vi "MSEncoder SubVI WfmCodeGen_PhaseScan.vi"(7 "Stepwise":i32, 8 "f2":ext, 9 "f1":ext, 10 "Scan time":ext, 11 "MSEncoder.lvclass":refnum<class "MSEncoder.lvclass">) -> (0 "WfmCode":u64[](array[numeric]), 1 "Actual Freq":dbl, 2 "Decyc":u64, 3 "1/Decyc":u32, 4 "error out":errorcluster)   [LabVIEW 2018, in "MSEncoder.lvclass"]
uses:
  MSEncoder.lvclass
  MSEncoder.lvclass/MSEncoder.ctl
panel:
  in  "High Res":bool
  in  "Interrupt":bool
  out "Phase Scan":cluster{"Scan time":ext, "Actual Freq":dbl}[](graph)
  out "Progress":dbl(slide) scale=0.0..0.05
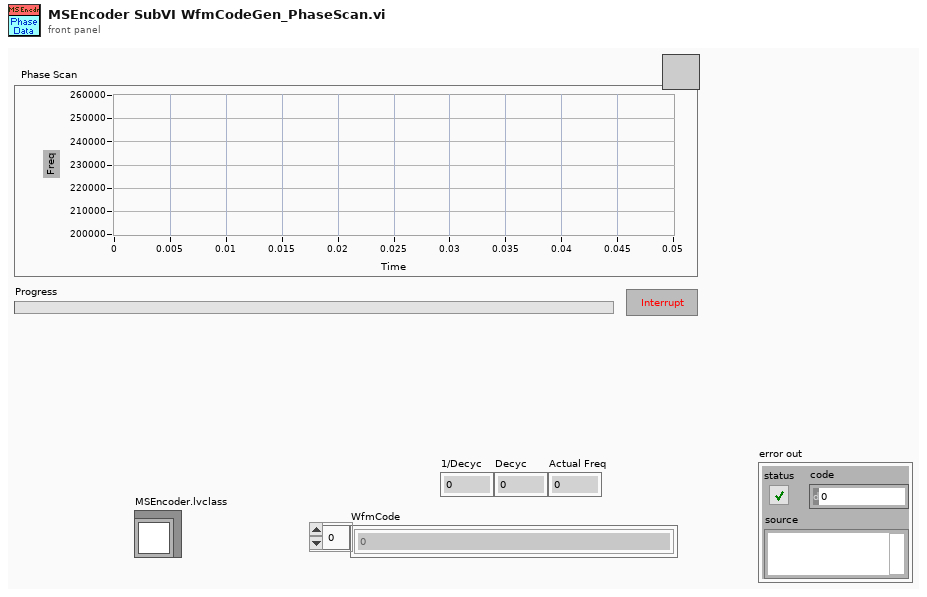
[diagram p1: front panel]
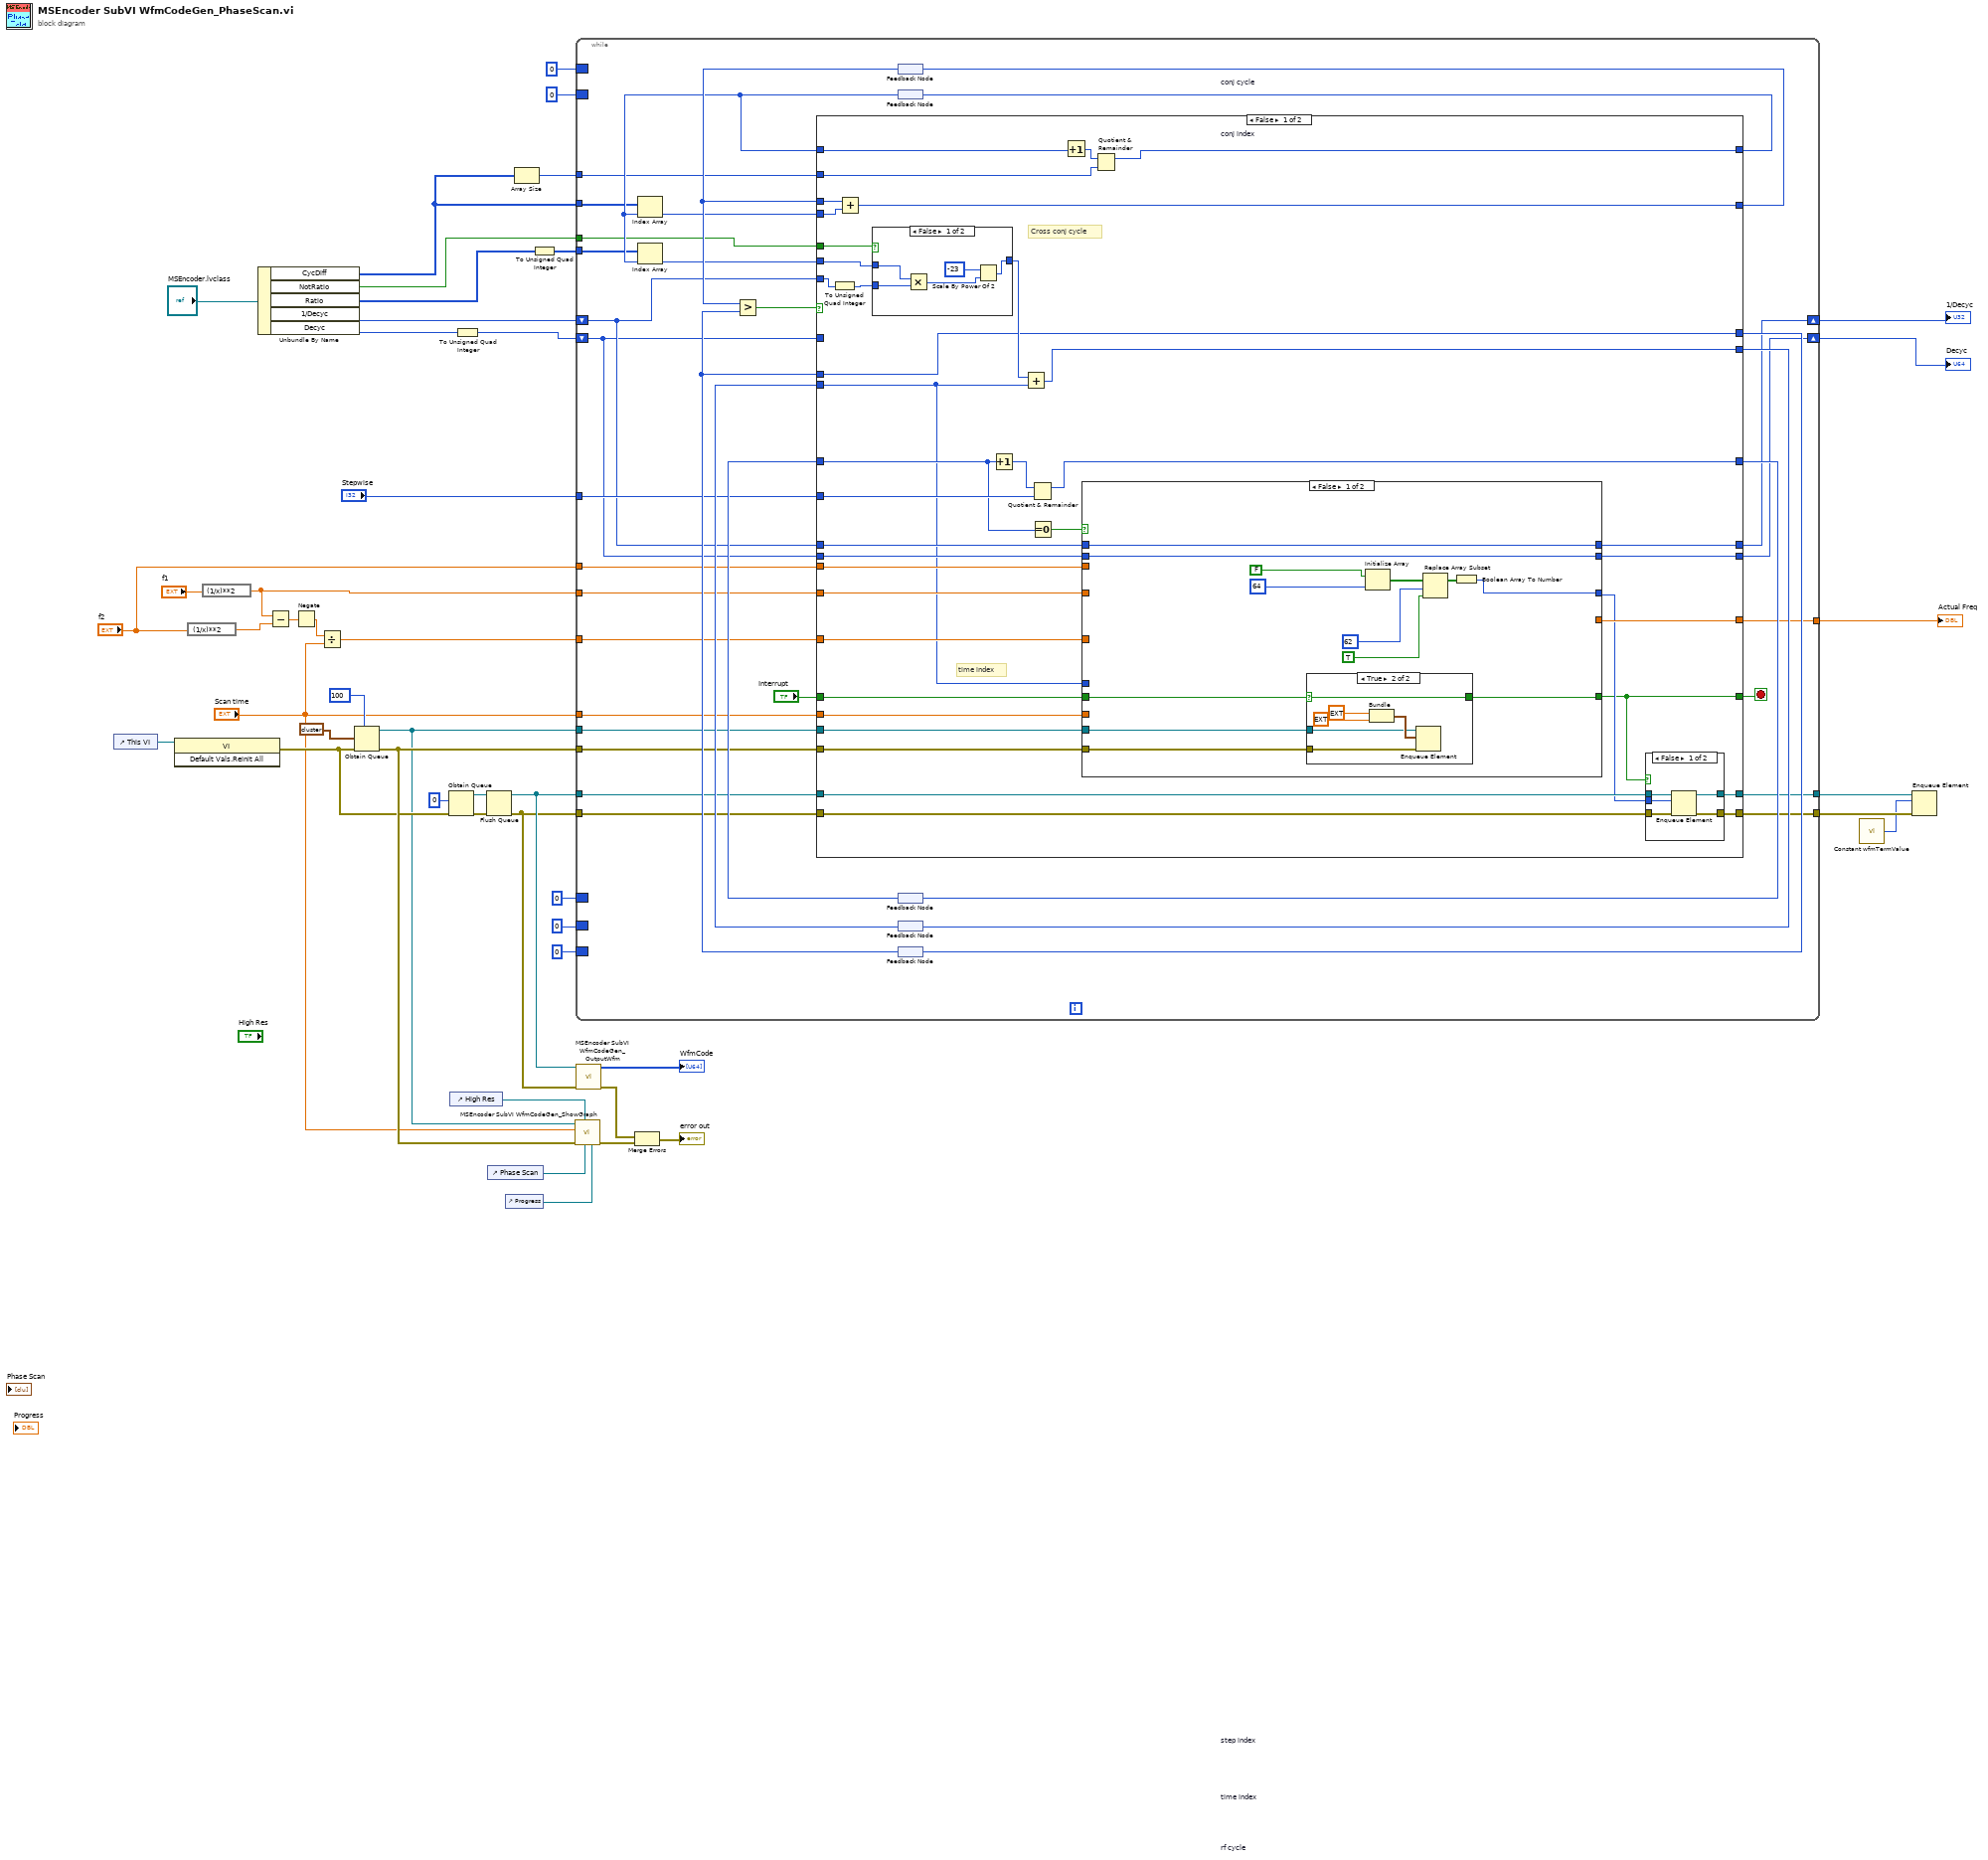
[diagram p0: block diagram]
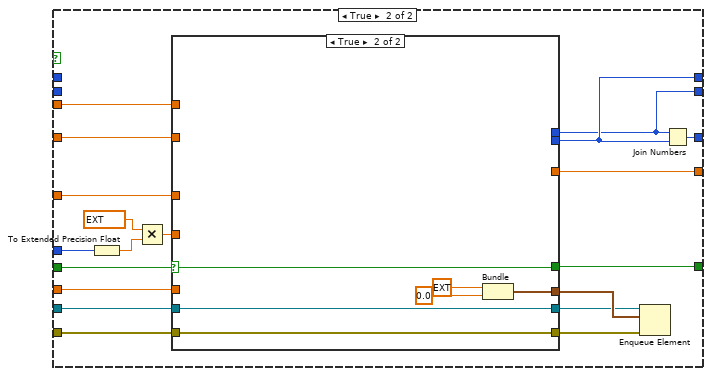
[diagram p5: hidden frame]
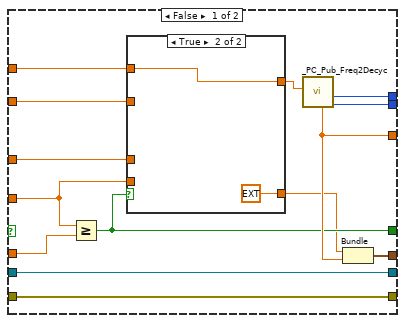
[diagram p6: hidden frame]
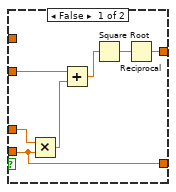
[diagram p7: hidden frame]
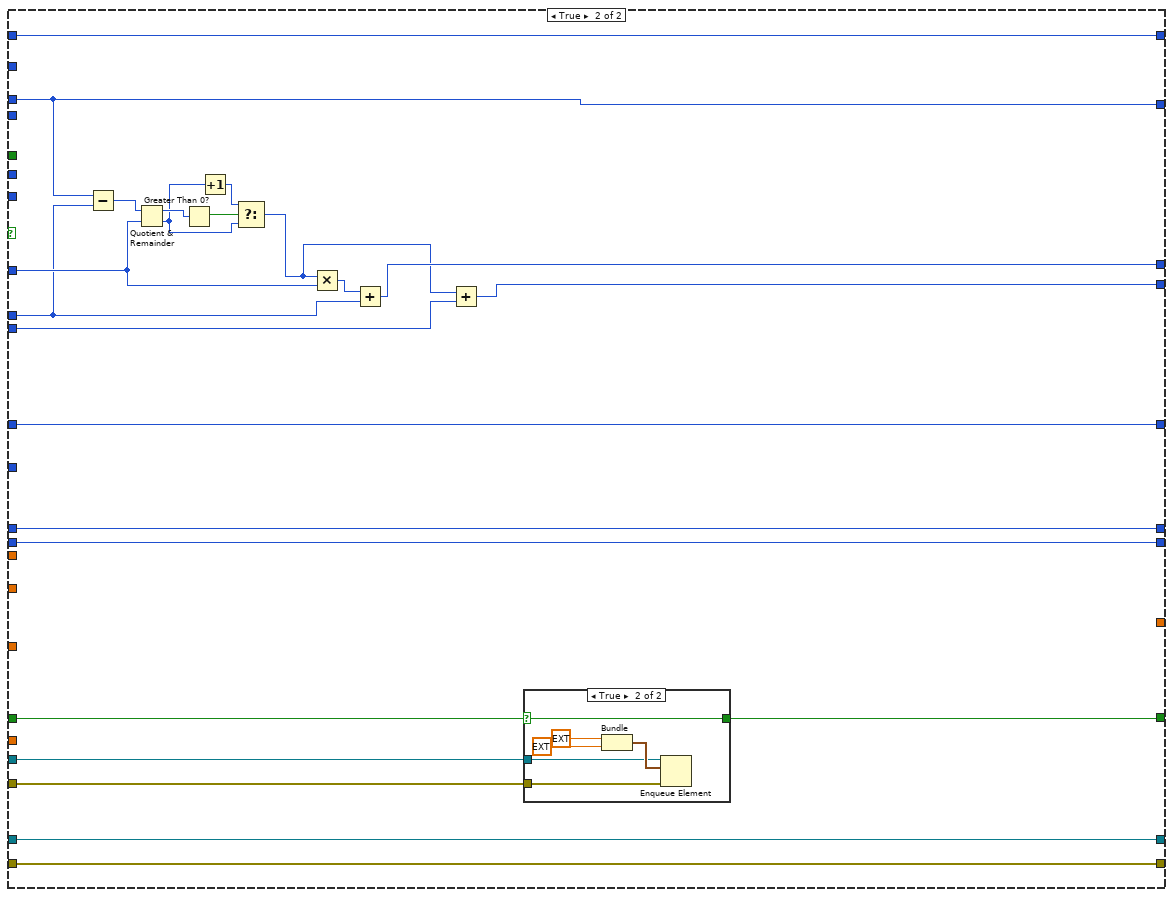
[diagram p8: hidden frame]
diagram:
  n1 = control-ref of="This VI"() -> (w6:refnum<vi>)
  n2 = invoke class="VI" method="Default Vals.Reinit All"(reference=w6) -> (error out=w5:errorcluster)  [unwired: 2 in, 2 out]
  n3 = expression code="(1/x)**2"("f2") -> (w42:ext)
  n4 = expression code="(1/x)**2"("f1") -> (w41:ext)
  n5 = Unbundle By Name("MSEncoder.lvclass") -> ("CycDiff"=w25:u64[], "NotRatio"=w24:bool, "Ratio"=w44:u16[], "1/Decyc"=w31:u32, "Decyc"=w30:u32)
  n6 = Subtract(x=w41, y=w42) -> (x-y=w40:ext)
  n7 = Negate(x=w40) -> (-x=w38:ext)
  n8 = Divide(x=w38, y="Scan time") -> (x/y=w39:ext)
  n9 = Obtain Queue(max queue size (-1, unlimited)=100, element data type=cluster{ext, "Amp2":ext} {0.0, "Amp2"=0.0} ("element"), error in (no error)=w5) -> (queue out=w2:refnum<queue>, error out=w13:errorcluster)  [unwired: 2 in, 1 out]
  n10 = Obtain Queue(element data type=u64 0, error in (no error)=w5) -> (queue out=w20:refnum<queue>, error out=w21:errorcluster)  [unwired: 3 in, 1 out]
  n11 = control-ref of="High Res"() -> (w1:refnum<vi>)
  n12 = To Unsigned Quad Integer(1:w30) -> (0:w26:u64)
  n13 = Flush Queue(queue=w20, error in (no error)=w21) -> (queue out=w16:refnum<queue>, error out=w15:errorcluster)  [unwired: 1 out]
  n14 = control-ref of="Phase Scan"() -> (w12:refnum<vi>)
  n15 = control-ref of="Progress"() -> (w11:refnum<vi>)
  n16 = Array Size(array=w25) -> (size(s)=w46:i32)
  n17 = To Unsigned Quad Integer(1:w44) -> (0:w27:u64[])
  n18 = call "MSEncoder SubVI WfmCodeGen_ShowGraph.vi"("progress refnum"=w11, "system graph refnum"=w12, "Graph Display"=w1, "error in (no error)"=w13, "X Scale.Range:Maximum"="Scan time", "Display queue in"=w2) -> ("error out"=w9:errorcluster)  [unwired: 5 in]
  n19 = while {
    tunnel: w25 -> [w78]
    tunnel: "Stepwise" -> [w68]
    border: u64 0 -> [_]
    border: u64 0 -> [_]
    tunnel: w46 -> [w74]
    border: u64 0 -> [_]
    tunnel: w41 -> [w64]
    shift-right: [w59] -> w32
    shift-left: w26 -> [w61]
    shift-right: [w60] -> w33
    shift-left: w31 -> [w62]
    tunnel: w27 -> [w77]
    tunnel: w39 -> [w65]
    tunnel: "Scan time" -> [w66]
    tunnel: "f2" -> [w63]
    tunnel: w2 -> [w57]
    tunnel: w13 -> [w56]
    border: 0 -> [_]
    border: 0 -> [_]
    tunnel: [w55] -> w34
    tunnel: w24 -> [w53]
    tunnel: w16 -> [w52]
    tunnel: w15 -> [w51]
    tunnel: [w50] -> w19
    tunnel: [w49] -> w18
    stop <- w58 stop-if-true
    n20 = feedback #1 "conj cycle"() -> (w82:u64)
    n21 = feedback #2 "conj index"() -> (w79:i32)
    n22 = Index Array(array=w78, index=w79) -> (element=w75:u64)
    n23 = Index Array(array=w77, index=w79) -> (element=w76:u64)
    n24 = feedback #3 "step index"() -> (w80:i32)
    n25 = feedback #4 "time index"() -> (w70:u64)
    n26 = feedback #5 "rf cycle"() -> (w81:u64)
    n27 = Greater?(x=w82, y=w81) -> (0:w54:bool)
    n28 = case shown="False" w54 {
      tunnel: w76 -> [w114 _]
      tunnel: w75 -> [w120 _]
      tunnel: w82 -> [w119 w215]
      tunnel: w61 -> [_ w214]
      tunnel: w81 -> [w91 w213]
      tunnel: w74 -> [w116 _]
      tunnel: [w118 w215] -> w73
      tunnel: w62 -> [w113 _]
      tunnel: w79 -> [w109 w224]
      tunnel: [w115 w224] -> w72
      tunnel: [w104 w220] -> w71
      tunnel: w70 -> [w93 w223]
      tunnel: [w91 w221] -> w69
      tunnel: w68 -> [w112 _]
      tunnel: [w111 w217] -> w67
      tunnel: w80 -> [w110 w217]
      tunnel: w66 -> [w108 _]
      tunnel: w65 -> [w107 _]
      tunnel: w64 -> [w106 _]
      tunnel: w63 -> [w105 _]
      tunnel: w62 -> [w103 w219]
      tunnel: w61 -> [w102 w218]
      tunnel: [w101 w219] -> w60
      tunnel: [w100 w218] -> w59
      tunnel: [w83 w204] -> w58
      tunnel: w57 -> [w99 w203]
      tunnel: w56 -> [w98 w202]
      tunnel: [w97 _] -> w55
      tunnel: w53 -> [w90 _]
      tunnel: w52 -> [w89 w207]
      tunnel: w51 -> [w88 w206]
      tunnel: [w86 w207] -> w50
      tunnel: [w85 w206] -> w49
      tunnel: "Interrupt" -> [w84 w205]
      frame False {
        # "time index"
        # "Cross conj cycle"
        n29 = To Unsigned Quad Integer(1:w113) -> (0:w96:u64)
        n30 = Add(x=w119, y=w120) -> (x+y=w118:u64)
        n31 = case shown="False" w90 {
          tunnel: w114 -> [w130 w133]
          tunnel: w96 -> [w128 _]
          tunnel: [w129 w133] -> w92
          frame False {
            n32 = Multiply(x=w130, y=w128) -> (x*y=w132:u64)
            n33 = Scale By Power Of 2(n=i16 -23, x=w132) -> (x*2^n=w129:u64)
          }
          frame True {
          }
        }
        n34 = Increment(x=w110) -> (x+1=w95:i32)
        n35 = Add(x=w92, y=w93) -> (x+y=w104:u64)
        n36 = Quotient & Remainder(x=w95, y=w112) -> (x-y*floor(x/y)=w111:i32)  [unwired: 1 out]
        n37 = Equal To 0?(x=w110) -> (x = 0?=w94:bool)
        n38 = Increment(x=w109) -> (x+1=w117:i32)
        n39 = case shown="False" w94 {
          tunnel: w105 -> [_ w172]
          tunnel: w106 -> [_ w171]
          tunnel: w108 -> [_ w165]
          tunnel: w107 -> [_ w170]
          tunnel: [w140 w169] -> w87
          tunnel: w93 -> [_ w166]
          tunnel: [w138 w161] -> w101
          tunnel: [w139 w160] -> w100
          tunnel: w103 -> [w138 _]
          tunnel: w102 -> [w139 _]
          tunnel: [w136 w159] -> w83
          tunnel: w99 -> [w135 w156]
          tunnel: w98 -> [w134 w154]
          tunnel: [_ w162] -> w97
          tunnel: w84 -> [w137 w158]
          frame False {
            n40 = case shown="True" w137 {
              selector: w137 -> [w147 w148]
              tunnel: w135 -> [_ w150]
              tunnel: w134 -> [_ w149]
              tunnel: [w147 w148] -> w136
              frame False {
              }
              frame True {
                n41 = Bundle(ext -1.0, ext 0.0) -> (w153:cluster{ext, ext})  [unwired: 1 in]
                n42 = Enqueue Element(queue=w150, element=w153, error in (no error)=w149) -> ()  [unwired: 1 in, 3 out]
              }
            }
            n43 = Initialize Array(FALSE, 64 ("dimension size")) -> (w144:bool[])
            n44 = Replace Array Subset(array=w144, new element=TRUE, index=62) -> (w141:bool[])
            n45 = Boolean Array To Number(Boolean array=w141) -> (number=w140:u64)
          }
          frame True {
            n46 = To Extended Precision Float(1:w166) -> (0:w167:ext)
            n47 = Multiply(x=ext 2.5e-08, y=w167) -> (x*y=w164:ext)
            n48 = case shown="True" w158 {
              selector: w158 -> [_ w201]
              tunnel: w172 -> [w185 _]
              tunnel: w171 -> [w184 _]
              tunnel: w170 -> [w183 _]
              tunnel: w165 -> [w182 _]
              tunnel: w164 -> [w181 _]
              tunnel: [w180 w198] -> w163
              tunnel: [w179 _] -> w162
              tunnel: [w178 _] -> w161
              tunnel: [w177 _] -> w160
              tunnel: [w176 w201] -> w159
              tunnel: [w175 w197] -> w157
              tunnel: w156 -> [w175 w197]
              tunnel: [w174 w196] -> w155
              tunnel: w154 -> [w174 w196]
              frame False {
                n49 = Greater Or Equal?(x=w181, y=w182) -> (x >= y?=w176:bool)
                n50 = case shown="True" w176 {
                  tunnel: [w190 w195] -> w186
                  tunnel: w185 -> [_ w195]
                  tunnel: w184 -> [w189 _]
                  tunnel: w183 -> [w188 _]
                  tunnel: w181 -> [w187 _]
                  tunnel: [w187 ext -2.0] -> w173
                  frame False {
                    n51 = Multiply(x=w188, y=w187) -> (x*y=w193:ext)
                    n52 = Add(x=w189, y=w193) -> (x+y=w192:ext)
                    n53 = Square Root(x=w192) -> (sqrt(x)=w191:ext)
                    n54 = Reciprocal(x=w191) -> (1/x=w190:ext)
                  }
                  frame True {
                  }
                }
                n55 = call "_PC_Pub_Freq2Decyc.vi"("Freq"=w186) -> ("(1/Decyc)*2^8"=w178:u32, "Decyc*2^32"=w177:u32, "Actual Freq"=w179:dbl)  [unwired: 4 in, 2 out]
                n56 = Bundle(w173, "Actual Freq"=w179) -> (w180:cluster{ext, "Actual Freq":dbl})  [unwired: 1 in]
              }
              frame True {
                n57 = Bundle(ext -1.0, 0.0) -> (w198:cluster{ext, dbl})  [unwired: 1 in]
              }
            }
            n58 = Enqueue Element(queue=w157, element=w163, error in (no error)=w155) -> ()  [unwired: 1 in, 3 out]
            n59 = Join Numbers(hi=w160, lo=w161) -> ((hi.lo)=w169:u64)
          }
        }
        n60 = Quotient & Remainder(x=w117, y=w116) -> (x-y*floor(x/y)=w115:i32)  [unwired: 1 out]
        n61 = case shown="False" w83 {
          tunnel: w89 -> [w125 w127]
          tunnel: w88 -> [w124 w126]
          tunnel: w87 -> [w123 _]
          tunnel: [w122 w127] -> w86
          tunnel: [w121 w126] -> w85
          frame False {
            n62 = Enqueue Element(queue=w125, element=w123, error in (no error)=w124) -> (queue out=w122:refnum<queue>, error out=w121:errorcluster)  [unwired: 1 in, 1 out]
          }
          frame True {
          }
        }
      }
      frame True {
        n63 = Subtract(x=w215, y=w213) -> (x-y=w216:u64)
        n64 = Quotient & Remainder(x=w216, y=w214) -> (x-y*floor(x/y)=w212:u64, floor(x/y)=w209:u64)
        n65 = Greater Than 0?(x=w212) -> (x > 0?=w211:bool)
        n66 = Increment(x=w209) -> (x+1=w210:u64)
        n67 = Select(t=w210, s=w211, f=w209) -> (s? t:f=w208:u64)
        n68 = Multiply(x=w208, y=w214) -> (x*y=w222:u64)
        n69 = Add(x=w222, y=w213) -> (x+y=w221:u64)
        n70 = Add(x=w208, y=w223) -> (x+y=w220:u64)
        n71 = case shown="True" w205 {
          selector: w205 -> [w225 w226]
          tunnel: w203 -> [_ w228]
          tunnel: w202 -> [_ w227]
          tunnel: [w225 w226] -> w204
          frame False {
          }
          frame True {
            n72 = Bundle(ext -1.0, ext 0.0) -> (w231:cluster{ext, ext})  [unwired: 1 in]
            n73 = Enqueue Element(queue=w228, element=w231, error in (no error)=w227) -> ()  [unwired: 1 in, 3 out]
          }
        }
      }
    }
    n74 = feedback-in #1(w73) -> ()
    n75 = feedback-in #2(w72) -> ()
    n76 = feedback-in #3(w67) -> ()
    n77 = feedback-in #4(w71) -> ()
    n78 = feedback-in #5(w69) -> ()
  }
  "1/Decyc" <- w33
  "Decyc" <- w32
  "Actual Freq" <- w34
  n79 = call "MSEncoder SubVI WfmCodeGen_OutputWfm.vi"("error in (no error)"=w15, "calc wfm queue"=w16) -> ("error out"=w10:errorcluster, "WfmCode"=→"WfmCode":u64[])  [unwired: 8 in]
  n80 = Merge Errors(w10, w9) -> (→"error out":errorcluster)
  n81 = call "Constant wfmTermValue.vi"() -> ("wfm end value"=w17:u64)
  n82 = Enqueue Element(queue=w19, element=w17, error in (no error)=w18) -> ()  [unwired: 1 in, 3 out]
